vi "NI VeriStand - Load Macro.vi"(8 "error in (no error)":errorcluster, 10 "File path":path, 11 "MacroPlayer in":T1) -> (0 "error out":errorcluster, 3 "MacroPlayer  out":T1)   [LabVIEW 2020, in "NI_VS MacroPlayerAPI.lvlib"]
doc: "Loads a previously recorded macro (.nivsmacro) file for playback. You can use the Macro Recorder VIs or the Macro Recorder tool in NI VeriStand to create macro files."
uses:
  <vilib>/NI VeriStand/Execution/MacroPlayer/NI_VS MacroPlayerAPI.lvlib
  <vilib>/NI VeriStand/Execution/MacroPlayer/MacroPlayerAPI.ctl
  NationalInstruments.VeriStand.ClientAPI
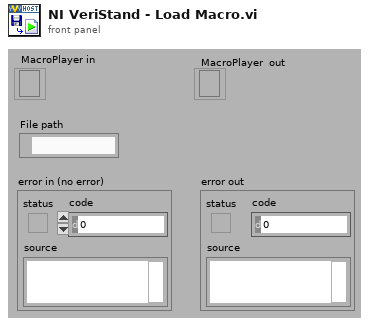
[diagram p1: front panel]
types:
  T1 = typedef "NI_VS MacroPlayerAPI.lvlib/MacroPlayerAPI.ctl" = refnum<k24>
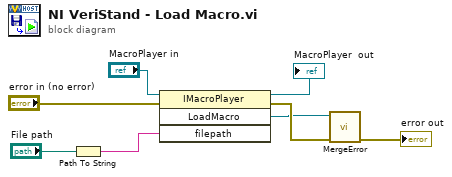
[diagram p0: block diagram]
diagram:
  n1 = Path To String(path="File path") -> (string=w1:string)
  n2 = invoke class="IMacroPlayer" method="LoadMacro"(reference="MacroPlayer in", error in="error in (no error)", "filepath"=w1) -> (reference out=→"MacroPlayer  out":T1, error out=w4:errorcluster, "LoadMacro"=w3:refnum<k24>)  [unwired: 1 in, 1 out]
  n3 = call <vilib>:"MergeError.vi"("error in (no error)"=w4, "Error"=w3) -> ("error out"=→"error out":errorcluster)  [unwired: 9 out]
